vi "LightFieldBackgroundFileName.vi"(8 "error in":errorcluster, 10 "File Exists":bool, 11 "FileName":string) -> (0 "error out":errorcluster)   [LabVIEW 2018]
uses:
  user32.dll
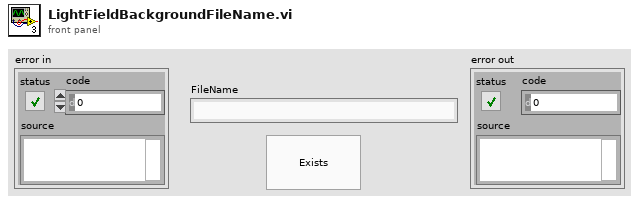
[diagram p1: front panel]
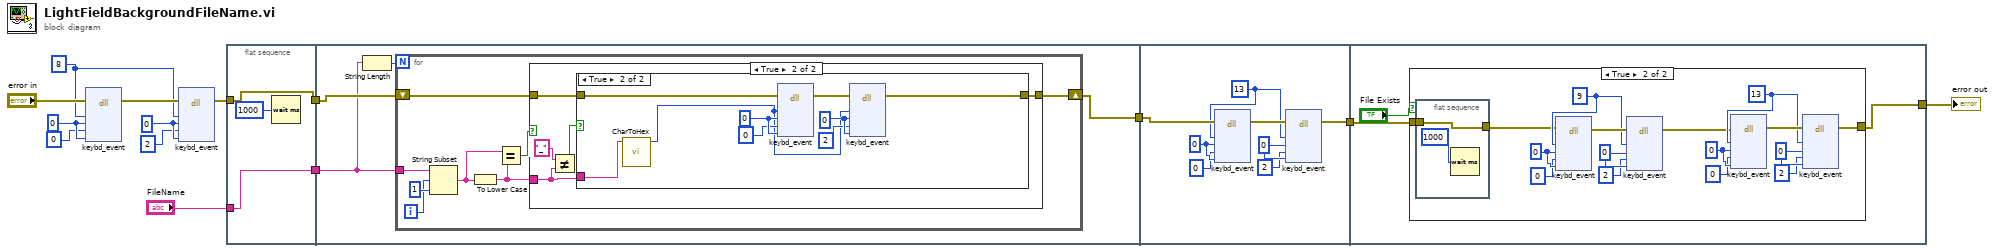
[diagram p0: block diagram]
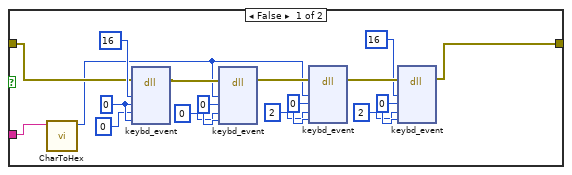
[diagram p2: hidden frame]
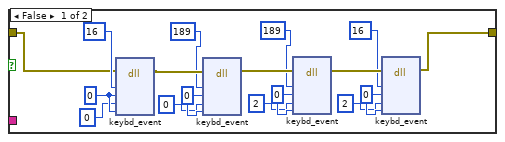
[diagram p3: hidden frame]
diagram:
  w8 = 8
  w12 = u8 0 ("bScan")
  w13 = u8 0 ("bScan")
  n1 = dll-call lib="user32.dll" fn="keybd_event"(error in="error in", "bVk"=w8, "bScan"=w13, "dwFlags"=0, "dwExtraInfo"=w13) -> (error out=w14:errorcluster)  [unwired: 7 in, 1 out]
  n2 = dll-call lib="user32.dll" fn="keybd_event"(error in=w14, "bVk"=w8, "bScan"=w12, "dwFlags"=2, "dwExtraInfo"=w12) -> (error out=w7:errorcluster)  [unwired: 7 in, 1 out]
  n3 = flat-sequence {
    tunnel: w7 -> [w16]
    tunnel: "FileName" -> [w15]
    tunnel: [w16] -> w5
    tunnel: [w15] -> w4
    tunnel: w5 -> [w20]
    tunnel: w4 -> [w19]
    tunnel: [w18] -> w3
    tunnel: w3 -> [w84]
    tunnel: [w85] -> w2
    tunnel: w2 -> [w87]
    tunnel: [w86] -> w1
    frame #0 {
      n4 = Wait (ms)(milliseconds to wait=u32 1000) -> ()  [unwired: 1 out]
    }
    frame #1 {
      n5 = String Length(string=w19) -> (length=w21:i32)
      n6 = for {
        N: w21 -> [_]
        shift-right: [w25] -> w18
        shift-left: w20 -> [w29]
        tunnel: w19 -> [w28]
        i -> [w26]
        n7 = String Subset(string=w28, offset (0)=w26, length (rest)=1 ("length (rest)")) -> (substring=w24:string)
        n8 = To Lower Case(string=w24) -> (all lower case string=w22:string)
        n9 = Equal?(x=w24, y=w22) -> (x = y?=w23:bool)
        n10 = case shown="True" w23 {
          tunnel: w29 -> [w33 w51]
          tunnel: [w32 w50] -> w25
          tunnel: w22 -> [w31 w47]
          frame False {
            w42 = u8 0 ("bScan")
            w40 = u8 0 ("bScan")
            w38 = u8 0 ("bScan")
            w35 = u8 0 ("bScan")
            n11 = call "CharToHex.vi"("Character"=w31) -> ("Hex"=w30:i32)  [unwired: 10 in]
            n12 = dll-call lib="user32.dll" fn="keybd_event"(error in=w33, "bVk"=16, "bScan"=w42, "dwFlags"=0, "dwExtraInfo"=w42) -> (error out=w45:errorcluster)  [unwired: 7 in, 1 out]
            n13 = dll-call lib="user32.dll" fn="keybd_event"(error in=w45, "bVk"=w30, "bScan"=w40, "dwFlags"=0, "dwExtraInfo"=w40) -> (error out=w44:errorcluster)  [unwired: 7 in, 1 out]
            n14 = dll-call lib="user32.dll" fn="keybd_event"(error in=w44, "bVk"=w30, "bScan"=w38, "dwFlags"=2, "dwExtraInfo"=w38) -> (error out=w46:errorcluster)  [unwired: 7 in, 1 out]
            n15 = dll-call lib="user32.dll" fn="keybd_event"(error in=w46, "bVk"=16, "bScan"=w35, "dwFlags"=2, "dwExtraInfo"=w35) -> (error out=w32:errorcluster)  [unwired: 7 in, 1 out]
          }
          frame True {
            n16 = Not Equal?(x="_", y=w47) -> (x != y?=w49:bool)
            n17 = case shown="True" w49 {
              tunnel: w51 -> [w53 w77]
              tunnel: [w52 w75] -> w50
              tunnel: w47 -> [_ w70]
              frame False {
                w64 = u8 0 ("bScan")
                w61 = u8 0 ("bScan")
                w58 = u8 0 ("bScan")
                w55 = u8 0 ("bScan")
                n18 = dll-call lib="user32.dll" fn="keybd_event"(error in=w53, "bVk"=16, "bScan"=w64, "dwFlags"=0, "dwExtraInfo"=w64) -> (error out=w67:errorcluster)  [unwired: 7 in, 1 out]
                n19 = dll-call lib="user32.dll" fn="keybd_event"(error in=w67, "bVk"=189, "bScan"=w61, "dwFlags"=0, "dwExtraInfo"=w61) -> (error out=w66:errorcluster)  [unwired: 7 in, 1 out]
                n20 = dll-call lib="user32.dll" fn="keybd_event"(error in=w66, "bVk"=189, "bScan"=w58, "dwFlags"=2, "dwExtraInfo"=w58) -> (error out=w68:errorcluster)  [unwired: 7 in, 1 out]
                n21 = dll-call lib="user32.dll" fn="keybd_event"(error in=w68, "bVk"=16, "bScan"=w55, "dwFlags"=2, "dwExtraInfo"=w55) -> (error out=w52:errorcluster)  [unwired: 7 in, 1 out]
              }
              frame True {
                w73 = u8 0 ("bScan")
                w74 = u8 0 ("bScan")
                n22 = call "CharToHex.vi"("Character"=w70) -> ("Hex"=w69:i32)  [unwired: 10 in]
                n23 = dll-call lib="user32.dll" fn="keybd_event"(error in=w77, "bVk"=w69, "bScan"=w74, "dwFlags"=0, "dwExtraInfo"=w74) -> (error out=w76:errorcluster)  [unwired: 7 in, 1 out]
                n24 = dll-call lib="user32.dll" fn="keybd_event"(error in=w76, "bVk"=w69, "bScan"=w73, "dwFlags"=2, "dwExtraInfo"=w73) -> (error out=w75:errorcluster)  [unwired: 7 in, 1 out]
              }
            }
          }
        }
      }
    }
    frame #2 {
      w82 = 13
      w79 = u8 0 ("bScan")
      w81 = u8 0 ("bScan")
      n25 = dll-call lib="user32.dll" fn="keybd_event"(error in=w84, "bVk"=w82, "bScan"=w79, "dwFlags"=0, "dwExtraInfo"=w79) -> (error out=w83:errorcluster)  [unwired: 7 in, 1 out]
      n26 = dll-call lib="user32.dll" fn="keybd_event"(error in=w83, "bVk"=w82, "bScan"=w81, "dwFlags"=2, "dwExtraInfo"=w81) -> (error out=w85:errorcluster)  [unwired: 7 in, 1 out]
    }
    frame #3 {
      n27 = case shown="True" "File Exists" {
        tunnel: w87 -> [w89 w99]
        tunnel: [w89 w98] -> w86
        frame False {
        }
        frame True {
          w96 = 9
          w93 = u8 0 ("bScan")
          w95 = u8 0 ("bScan")
          w104 = 13
          w101 = u8 0 ("bScan")
          w103 = u8 0 ("bScan")
          n28 = flat-sequence {
            tunnel: w99 -> [w107]
            tunnel: [w107] -> w91
            frame #0 {
              n29 = Wait (ms)(milliseconds to wait=u32 1000) -> ()  [unwired: 1 out]
            }
          }
          n30 = dll-call lib="user32.dll" fn="keybd_event"(error in=w91, "bVk"=w96, "bScan"=w93, "dwFlags"=0, "dwExtraInfo"=w93) -> (error out=w97:errorcluster)  [unwired: 7 in, 1 out]
          n31 = dll-call lib="user32.dll" fn="keybd_event"(error in=w97, "bVk"=w96, "bScan"=w95, "dwFlags"=2, "dwExtraInfo"=w95) -> (error out=w90:errorcluster)  [unwired: 7 in, 1 out]
          n32 = dll-call lib="user32.dll" fn="keybd_event"(error in=w90, "bVk"=w104, "bScan"=w101, "dwFlags"=0, "dwExtraInfo"=w101) -> (error out=w105:errorcluster)  [unwired: 7 in, 1 out]
          n33 = dll-call lib="user32.dll" fn="keybd_event"(error in=w105, "bVk"=w104, "bScan"=w103, "dwFlags"=2, "dwExtraInfo"=w103) -> (error out=w98:errorcluster)  [unwired: 7 in, 1 out]
        }
      }
    }
  }
  "error out" <- w1
